vi "UI_Set_Initial_tabs_representation.vi"(2 "error in (no error)":errorcluster, 3 "Controls references":T1) -> (0 "error out":errorcluster)   [LabVIEW 2018, in "Tracker.lvlib"]
uses:
  Tracker.lvlib
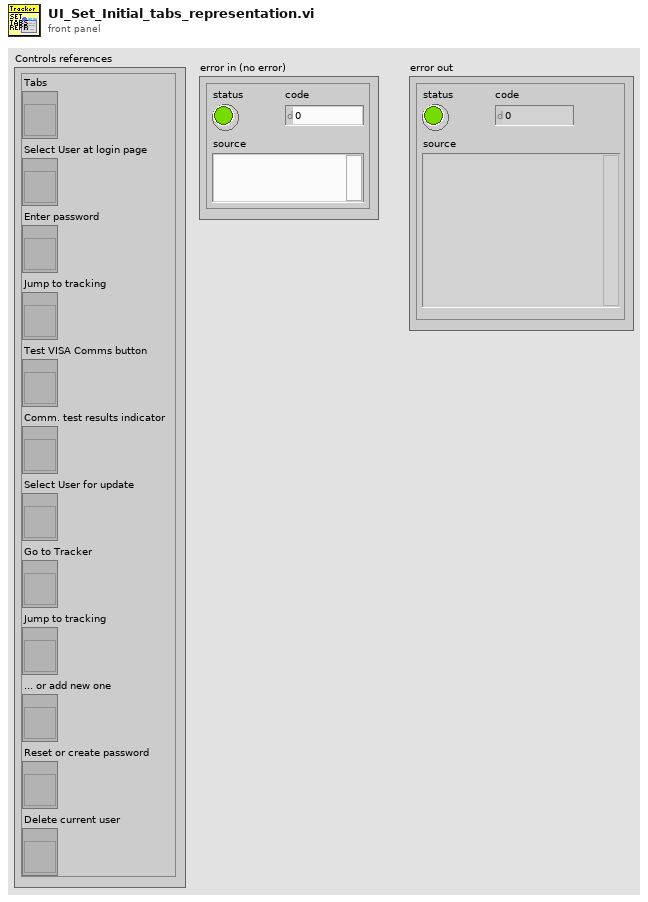
[diagram p1: front panel]
types:
  T1 = cluster{"Tabs":refnum<vi>, "Select User at login page":refnum<vi>, "Enter password":refnum<vi>, "Jump to tracking":refnum<vi>, "Test VISA Comms button":refnum<vi>, "Comm. test results indicator":refnum<vi>, "Select User for update":refnum<vi>, "Go to Tracker":refnum<vi>, "Jump to tracking":refnum<vi>, "... or add new one":refnum<vi>, "Reset or create password":refnum<vi>, "Delete current user":refnum<vi>}
  T2 = enum8{"Enabled", "Disabled", "Disabled and Grayed Out"}
  T3 = enum32{"Page Enabled", "Page Disabled", "Page Disabled & Grayed"}
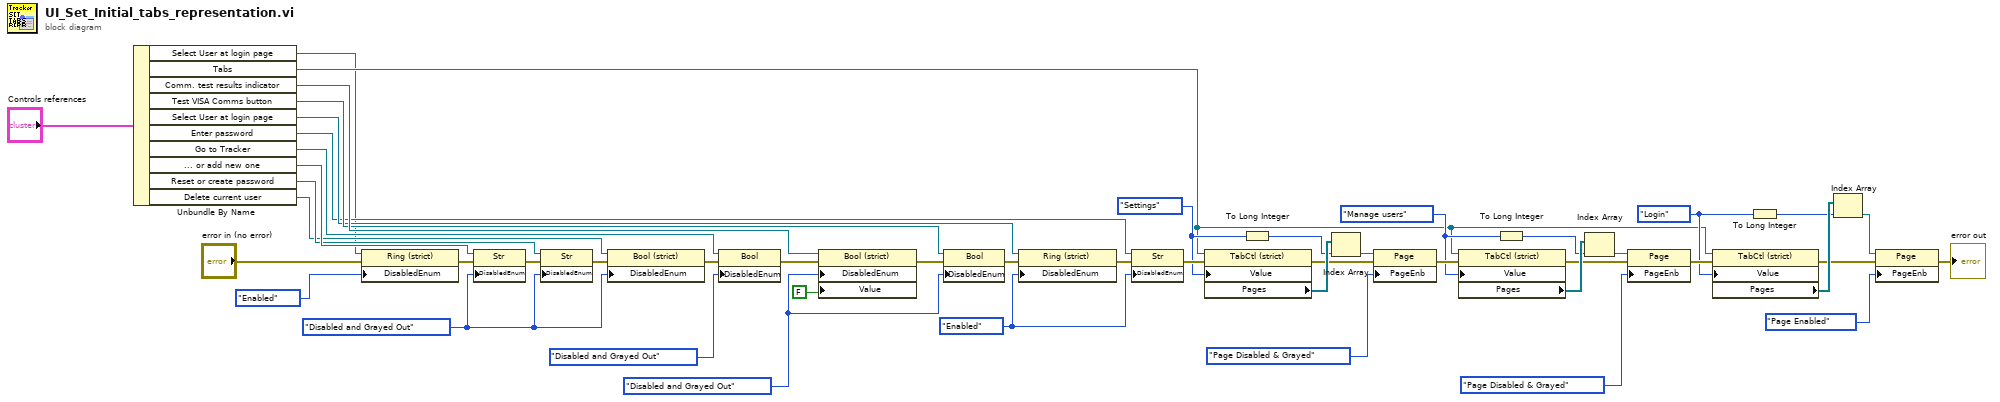
[diagram p0: block diagram]
diagram:
  w8 = T2."Disabled and Grayed Out" ("Disabled")
  w22 = T2."Disabled and Grayed Out" ("Disabled")
  w30 = enum32{"Login", "Settings", "Manage users"}."Login" ("Login tab")
  w44 = enum32{"Login", "Settings", "Manage users"}."Manage users" ("Login tab")
  w38 = enum32{"Login", "Settings", "Manage users"}."Settings" ("Login tab")
  w33 = T2."Enabled" ("Disabled")
  n1 = Unbundle By Name("Controls references") -> ("Select User at login page"=w2:refnum<vi>, "Tabs"=w20:refnum<vi>, "Comm. test results indicator"=w19:refnum<vi>, "Test VISA Comms button"=w18:refnum<vi>, "Select User at login page"=w17:refnum<vi>, "Enter password"=w16:refnum<vi>, "Go to Tracker"=w13:refnum<vi>, "... or add new one"=w7:refnum<vi>, "Reset or create password"=w6:refnum<vi>, "Delete current user"=w5:refnum<vi>)
  n2 = property class="Ring (strict)"(reference=w2, error in="error in (no error)", "DisabledEnum"=T2."Enabled" ("Disabled")) -> (error out=w4:errorcluster)  [unwired: 1 out]
  n3 = property class="Str"(reference=w7, error in=w4, "DisabledEnum"=w8) -> (error out=w11:errorcluster)  [unwired: 1 out]
  n4 = property class="Str"(reference=w6, error in=w11, "DisabledEnum"=w8) -> (error out=w10:errorcluster)  [unwired: 1 out]
  n5 = property class="Bool (strict)"(reference=w5, error in=w10, "DisabledEnum"=w8) -> (error out=w9:errorcluster)  [unwired: 1 out]
  n6 = property class="Bool"(reference=w13, error in=w9, "DisabledEnum"=T2."Disabled and Grayed Out" ("Disabled")) -> (error out=w15:errorcluster)  [unwired: 1 out]
  n7 = property class="Bool (strict)"(reference=w19, error in=w15, "DisabledEnum"=w22, "Value"=FALSE) -> (error out=w23:errorcluster)  [unwired: 1 out]
  n8 = property class="Bool"(reference=w18, error in=w23, "DisabledEnum"=w22) -> (error out=w24:errorcluster)  [unwired: 1 out]
  n9 = property on="Property Node" class="Ring (strict)"(reference=w17, error in=w24, "DisabledEnum"=w33) -> (error out=w32:errorcluster)  [unwired: 1 out]
  n10 = property on="Property Node" class="Str"(reference=w16, error in=w32, "DisabledEnum"=w33) -> (error out=w47:errorcluster)  [unwired: 1 out]
  n11 = property on="Property Node" class="TabCtl (strict)"(reference=w20, error in=w47, "Value"=w38) -> (error out=w35:errorcluster, "Pages"=w39:refnum<vi>[])  [unwired: 1 out]
  n12 = To Long Integer(number=w38) -> (32bit integer=w37:i32)
  n13 = Index Array(array=w39, index=w37) -> (element=w36:refnum<vi>)
  n14 = property class="Page"(reference=w36, error in=w35, "PageEnb"=T3."Page Disabled & Grayed" ("Page Enabled State")) -> (error out=w48:errorcluster)  [unwired: 1 out]
  n15 = property on="Property Node" class="TabCtl (strict)"(reference=w20, error in=w48, "Value"=w44) -> (error out=w41:errorcluster, "Pages"=w45:refnum<vi>[])  [unwired: 1 out]
  n16 = To Long Integer(number=w44) -> (32bit integer=w43:i32)
  n17 = Index Array(array=w45, index=w43) -> (element=w42:refnum<vi>)
  n18 = property class="Page"(reference=w42, error in=w41, "PageEnb"=T3."Page Disabled & Grayed" ("Page Enabled State")) -> (error out=w46:errorcluster)  [unwired: 1 out]
  n19 = property on="Property Node" class="TabCtl (strict)"(reference=w20, error in=w46, "Value"=w30) -> (error out=w27:errorcluster, "Pages"=w31:refnum<vi>[])  [unwired: 1 out]
  n20 = To Long Integer(number=w30) -> (32bit integer=w29:i32)
  n21 = Index Array(array=w31, index=w29) -> (element=w28:refnum<vi>)
  n22 = property class="Page"(reference=w28, error in=w27, "PageEnb"=T3."Page Enabled" ("Page Enabled State")) -> (error out=→"error out":errorcluster)  [unwired: 1 out]
